vi "Listening Server Cases.vi"(7 "Listening Queue":refnum<queue>, 8 "error in (no error)":errorcluster, 9 "Data":variant, 10 "Command":string, 11 "LC Parser in":refnum<class "LC Parser.lvclass">) -> (0 "error out":errorcluster, 2 "Stop?":bool, 3 "LC Parser out":refnum<class "LC Parser.lvclass">)   [LabVIEW 2020, in "LC Parser.lvclass"]
doc: "Case structure with messages to listen for from the control panel. If more than the basic messages need to be handled, this should be overwritten by the child class."
uses:
  LC Parser.lvclass
  LC Parser.lvclass/LC Parser.ctl
  Sub VIs/Message Queue/test Message Queue.lvlib
  Sub VIs/Message Queue/Enqueue Message (Single).vi
  Controller/Generic Plugin.lvclass
  events/Process Stopped Cluster.ctl
  Z:/business/research/rxn_rover/Reaction Rover/Plugin Servers/Controller/Generic Plugin.lvclass
  <userlib>/Dynamic Reentrant/Type Defs/Message.ctl
  <userlib>/Dynamic Reentrant/Dynamic Reentrant.lvlib
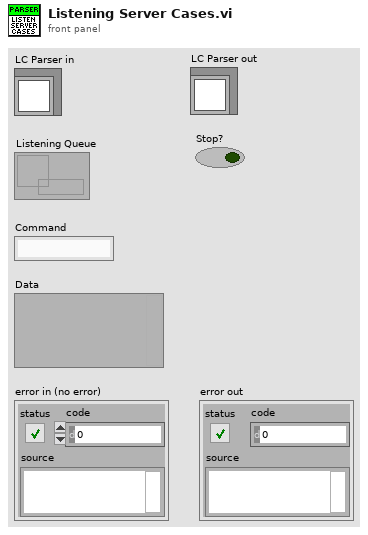
[diagram p1: front panel]
types:
  T1 = typedef "Process Stopped Cluster.ctl" = cluster{"Name":string, "Type":enum16{"Hardware", "Optimizer", "Analyzer"}}
  T2 = typedef "LC Parser.lvclass/LC Parser State.ctl" = cluster{"Data File":path, "Last Modified":timestamp, "Peak Data":cluster{"Time Stamp":timestamp, "Peaks":string[][]}, "Yield":dbl, "New File":bool}
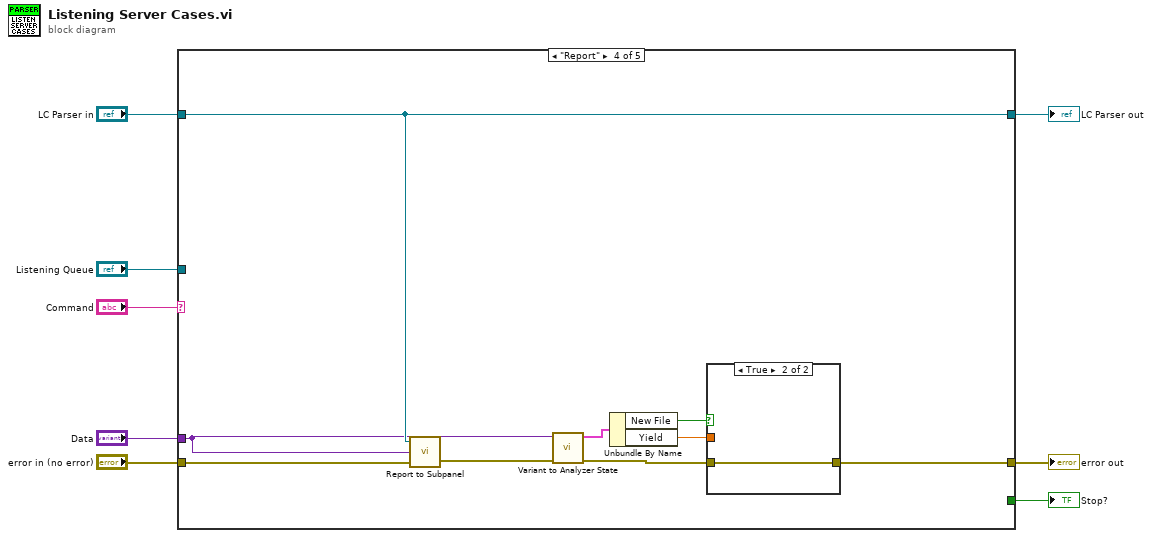
[diagram p0: block diagram]
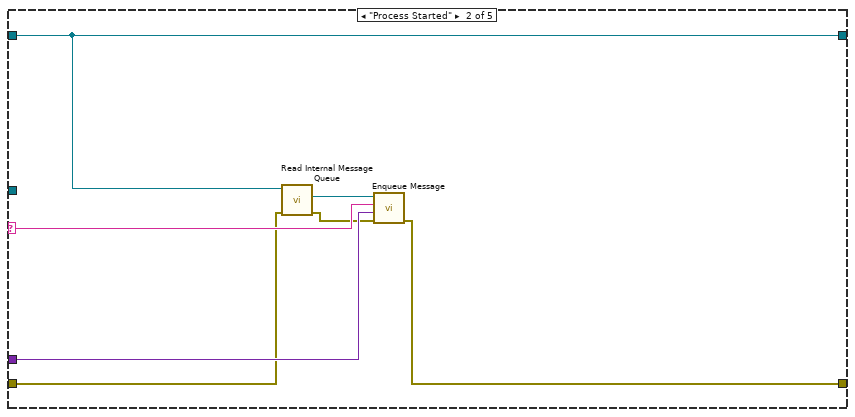
[diagram p3: hidden frame]
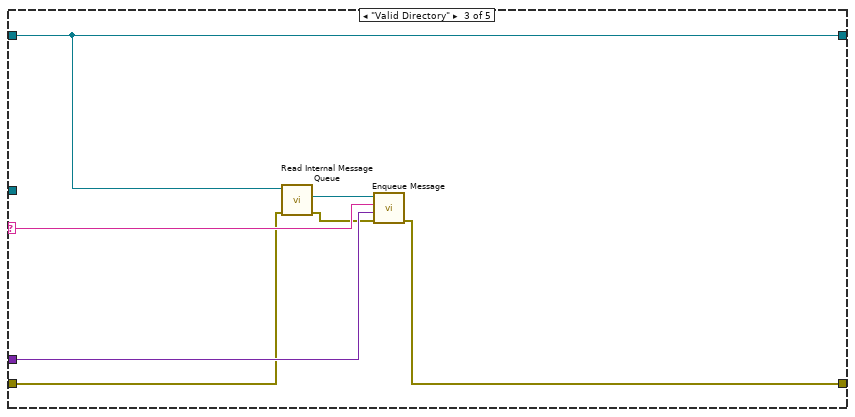
[diagram p4: hidden frame]
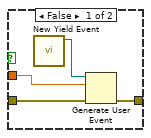
[diagram p5: hidden frame]
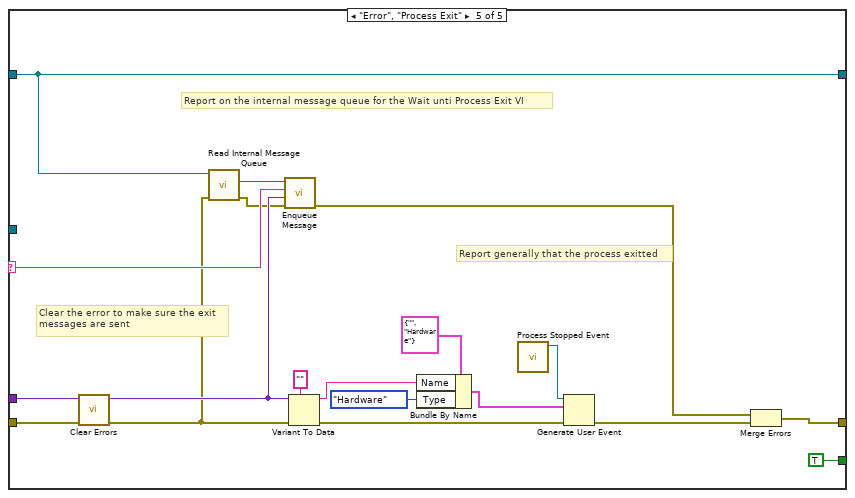
[diagram p6: hidden frame]
diagram:
  n1 = case shown="\"Report\"" "Command" {
    selector: "Command" -> [_ w17 w24 _ w47]
    tunnel: "error in (no error)" -> [w9 w11 w18 w33 w42]
    tunnel: [w9 w15 w22 w29 w45] -> w5
    tunnel: "LC Parser in" -> [w10 w13 w20 w32 w40]
    tunnel: [w10 w13 w20 w32 w40] -> w7
    tunnel: "Data" -> [_ w16 w23 w28 w46]
    tunnel: [_ _ _ _ TRUE] -> w6
    tunnel: "Listening Queue" -> [_ _ _ _ _]
    frame Default {
    }
    frame "Process Started" {
      n2 = call "Read Internal Message Queue.vi"("error in (no error)"=w11, "Generic Controller in"=w13) -> ("error out"=w12:errorcluster, "Internal Message Queue"=w14:refnum<queue>)  [unwired: 7 in, 1 out]
      n3 = call-poly "Enqueue Message.vi"("error in (no error)"=w12, "Message Data"=w16, "Message"=w17, "Message Queue"=w14) -> ("error out"=w15:errorcluster)  [unwired: 6 in, 1 out]
    }
    frame "Valid Directory" {
      n4 = call "Read Internal Message Queue.vi"("error in (no error)"=w18, "Generic Controller in"=w20) -> ("error out"=w19:errorcluster, "Internal Message Queue"=w21:refnum<queue>)  [unwired: 7 in, 1 out]
      n5 = call-poly "Enqueue Message.vi"("error in (no error)"=w19, "Message Data"=w23, "Message"=w24, "Message Queue"=w21) -> ("error out"=w22:errorcluster)  [unwired: 6 in, 1 out]
    }
    frame "Report" {
      n6 = call "Report to Subpanel.vi"("error in (no error)"=w33, "State"=w28, "controller in"=w32) -> ("error out"=w31:errorcluster)  [unwired: 1 out]
      n7 = call "Variant to Analyzer State.vi"("error in (no error)"=w31, "Message Data"=w28) -> ("error out"=w30:errorcluster, "Analyzer State"=w27:T2)  [unwired: 8 in]
      n8 = Unbundle By Name(w27) -> ("New File"=w25:bool, "Yield"=w26:dbl)
      n9 = case shown="True" w25 {
        tunnel: w30 -> [w36 w38]
        tunnel: [w35 w38] -> w29
        tunnel: w26 -> [w34 _]
        frame False {
          n10 = call "New Yield Event.vi"() -> ("New Yield"=w37:refnum<user-event>)  [unwired: 11 in]
          n11 = Generate User Event(user event=w37, event data cluster=w34, error in=w36) -> (error out=w35:errorcluster)  [unwired: 1 in, 1 out]
        }
        frame True {
        }
      }
    }
    frame "Error", "Process Exit" {
      # "Clear the error to make sure the exit\nmessages are sent"
      # "Report generally that the process exitted"
      # "Report on the internal message queue for the Wait unti Process Exit VI"
      n12 = call <vilib>:"Clear Errors.vi"("error in (no error)"=w42) -> ("error out"=w39:errorcluster)  [unwired: 5 in, 1 out]
      n13 = call "Read Internal Message Queue.vi"("error in (no error)"=w39, "Generic Controller in"=w40) -> ("error out"=w41:errorcluster, "Internal Message Queue"=w43:refnum<queue>)  [unwired: 7 in, 1 out]
      n14 = call-poly "Enqueue Message.vi"("error in (no error)"=w41, "Message Data"=w46, "Message"=w47, "Message Queue"=w43) -> ("error out"=w44:errorcluster)  [unwired: 6 in, 1 out]
      n15 = Variant To Data(error in=w39, type="", Variant=w46) -> (data=w49:string, error out=w53:errorcluster)
      n16 = Bundle By Name(cluster=T1 {"Name"="", "Type"=enum."Hardware"} ("Process Cluster"), "Name"=w49, "Type"=enum16{"Hardware", "Optimizer"}."Hardware") -> (w50:T1)
      n17 = call "Process Stopped Event.vi"() -> ("Process Stopped"=w55:refnum<user-event>)  [unwired: 11 in]
      n18 = Generate User Event(user event=w55, event data cluster=w50, error in=w53) -> (error out=w54:errorcluster)  [unwired: 1 in, 1 out]
      n19 = Merge Errors(w44, w54) -> (w45:errorcluster)
    }
  }
  "Stop?" <- w6
  "LC Parser out" <- w7
  "error out" <- w5
